vi "PWM Instrumentation Lab 1.vi"() -> ()   [LabVIEW 2020]
uses:
  <vilib>/MakerHub/LINX/Public/Utilities/Open Serial.vi
  <vilib>/MakerHub/LINX/Public/Peripherals/PWM/PWM Set Duty Cycle N Chans.vi
  <vilib>/MakerHub/LINX/LMH-LINX.lvlib
panel:
  out "Waveform Graph":dynamicdata(graph)
  in  "Offset":dbl=0.5
  in  "Amplitude":dbl=0.5
  out "Color Indicator":u32(colorbox)
  in  "R Phase":dbl caption="Phase"
  in  "G Phase":dbl caption="Phase"
  in  "B Phase":dbl caption="Phase"
  in  "Frequency":dbl=1.0
  in  "R":u8
  in  "G":u8
  in  "stop":bool
  in  "B":u8
  in  "Serial Port":refnum<visa-resource-name>="N/A"
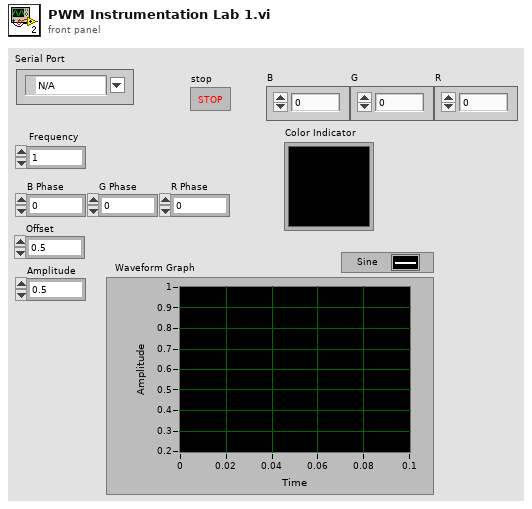
[diagram p1: front panel]
types:
  T1 = typedef "LMH-LINX.lvlib/LINX Ref.ctl" = cluster{"IO":T2, "Interface":T3, "LINX Device Config":T4}
  T2 = typedef "LMH-LINX.lvlib/Platform.ctl" = enum16{"Remote", "Local"}
  T3 = typedef "LMH-LINX.lvlib/Interface.ctl" = enum16{"Serial", "TCP"}
  T4 = typedef "LMH-LINX.lvlib/Device.lvlib/LINX Device Config.ctl" = cluster{"Interface":T3, "COM Port":refnum<visa-resource-name>, "TCP Configuration":T5, "Device Family":u8, "Device ID":u8, "Device Name":string, "TCP Ref":refnum<k5>, "Channels":T6}
  T5 = typedef "LMH-LINX.lvlib/Device.lvlib/TCP Config.ctl" = cluster{"IP Address":string, "Port":u16}
  T6 = typedef "LMH-LINX.lvlib/Channels.ctl" = cluster{"DI":u8[], "DO":u8[], "AI":u8[], "AO":u8[], "PWM":u8[], "QE":u8[], "UART":u8[], "I2C 2":u8[], "SPI":u8[], "CAN":u8[], "Servo":u8[], "AI Ref (V)":dbl, "AI Resolution (Bits)":u8, "AO Ref (V)":dbl, "AO Resolution (Bits)":u8}
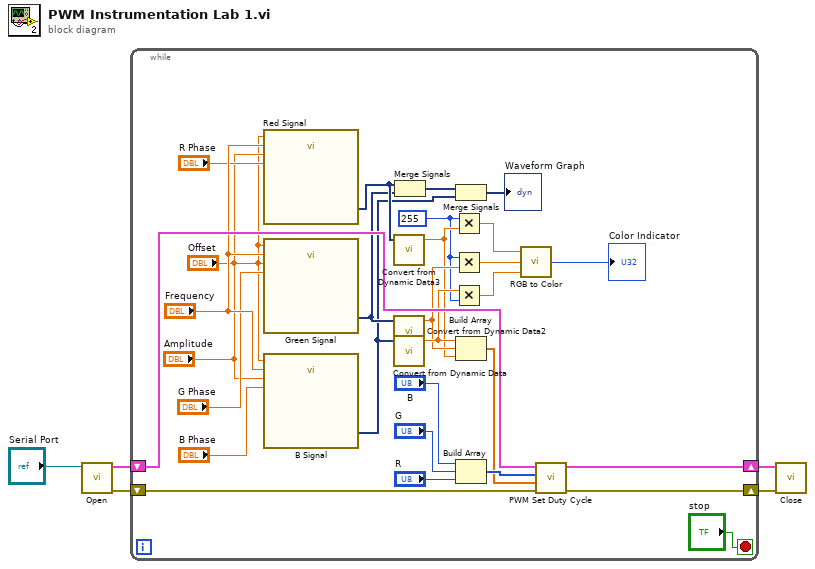
[diagram p0: block diagram]
diagram:
  n1 = call-poly <vilib>:"Open.vi"("Serial Port"="Serial Port") -> ("Error Out"=w2:errorcluster, "LINX Resource"=w4:T1)  [unwired: 8 in, 1 out]
  n2 = while {
    shift-right: [w33] -> w3
    shift-left: w4 -> [w34]
    shift-right: [w31] -> w1
    shift-left: w2 -> [w32]
    stop <- "stop" stop-if-true
    w7 = 255
    n3 = call "Red Signal"("Offset"="Offset", "Frequency"="Frequency", "Amplitude"="Amplitude", "Phase"="R Phase") -> ("Sine"=w12:dynamicdata)  [unwired: 10 in, 1 out]
    n4 = call "Green Signal"("Offset"="Offset", "Frequency"="Frequency", "Amplitude"="Amplitude", "Phase"="G Phase") -> ("Sine"=w10:dynamicdata)  [unwired: 10 in, 1 out]
    n5 = call "B Signal"("Offset"="Offset", "Frequency"="Frequency", "Amplitude"="Amplitude", "Phase"="B Phase") -> ("Sine"=w8:dynamicdata)  [unwired: 10 in, 1 out]
    n6 = call "Convert from Dynamic Data3"("Dynamic Data Type"=w12) -> ("Scalar"=w17:dbl)  [unwired: 3 in]
    n7 = call "Convert from Dynamic Data2"("Dynamic Data Type"=w10) -> ("Scalar"=w18:dbl)  [unwired: 3 in]
    n8 = call "Convert from Dynamic Data"("Dynamic Data Type"=w8) -> ("Scalar"=w20:dbl)  [unwired: 3 in]
    n9 = Merge Signals(w12, w10) -> (w11:dynamicdata)
    n10 = Multiply(x=w7, y=w17) -> (x*y=w16:dbl)
    n11 = Multiply(x=w7, y=w18) -> (x*y=w15:dbl)
    n12 = Multiply(x=w20, y=w7) -> (x*y=w19:dbl)
    n13 = Merge Signals(w11, w8) -> (→"Waveform Graph":dynamicdata)
    n14 = Build Array(w20, w18, w17) -> (w6:dbl[])
    n15 = Build Array("B", "G", "R") -> (w26:u8[])
    n16 = call <vilib>:"RGB to Color.vi"("B"=w19, "G"=w15, "R"=w16) -> ("Color"=→"Color Indicator":u32)
    n17 = call-poly <vilib>:"PWM Set Duty Cycle.vi"("Error In"=w32, "Duty Cycles"=w6, "PWM Channels"=w26, "LINX Resource"=w34) -> ("Error Out"=w31:errorcluster, "LINX Resource"=w33:T1)  [unwired: 6 in]
  }
  n18 = call <vilib>:"Close.vi"("Error In"=w1, "LINX Resource"=w3) -> ()  [unwired: 9 in, 1 out]
